vi "Dryer Status to Txt.vi"(11 "Status":T1) -> (3 "Ring Text.Text":string)   [LabVIEW 2009]
uses:
  Dryer Wilt/Dryer Status Ctrl.ctl
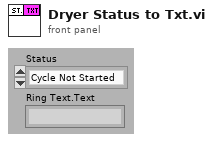
[diagram p1: front panel]
types:
  T1 = typedef "Dryer Status Ctrl.ctl" = enum16{"Cycle Not Started", "Cycle Running", "Paused", "Cycle Completed", "Eval Mode Entered", "Err"}
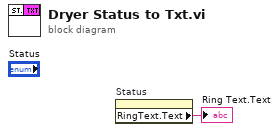
[diagram p0: block diagram]
diagram:
  n1 = property on="Status" class="Enum (strict)"() -> ("RingText.Text"=→"Ring Text.Text":string)  [unwired: 2 in, 2 out]
